vi "Passband_filter.vi"(8 "Lower bound":dbl, 9 "Upper bound":dbl, 11 "Array in":dbl[](array[numeric])) -> (3 "Array out":dbl[](array[numeric]))   [LabVIEW 2018]
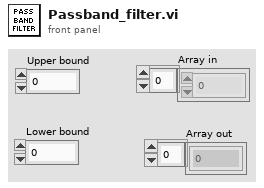
[diagram p1: front panel]
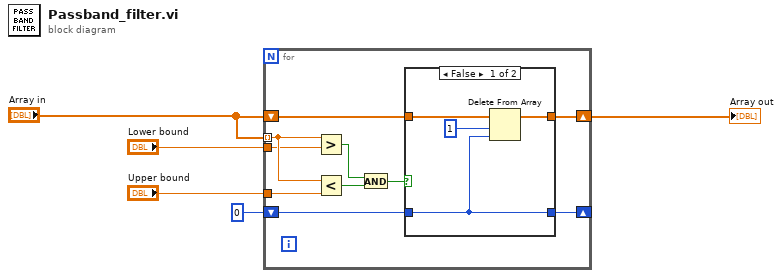
[diagram p0: block diagram]
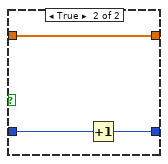
[diagram p2: hidden frame]
diagram:
  n1 = for {
    tunnel: "Array in" -> [w12] mode=indexing
    shift-right: [w10] -> w2
    shift-left: "Array in" -> [w11]
    shift-right: [w9] -> _
    shift-left: 0 -> [w8]
    tunnel: "Lower bound" -> [w7]
    tunnel: "Upper bound" -> [w6]
    n2 = Greater?(x=w12, y=w7) -> (0:w15:bool)
    n3 = Less?(x=w12, y=w6) -> (x < y?=w14:bool)
    n4 = And(x=w15, y=w14) -> (x .and. y?=w13:bool)
    n5 = case shown="False" w13 {
      tunnel: w11 -> [w17 w22]
      tunnel: [w19 w22] -> w10
      tunnel: [w16 w20] -> w9
      tunnel: w8 -> [w16 w21]
      frame False {
        n6 = Delete From Array(array=w17, length=1, index=w16) -> (array with subset deleted=w19:dbl[])  [unwired: 1 out]
      }
      frame True {
        n7 = Increment(x=w21) -> (x+1=w20:i32)
      }
    }
  }
  "Array out" <- w2
